vi "Test Digital Input.vi"(8 "error in":errorcluster, 10 "TestCase in":refnum<class "Scan Engine Scripting API Modules.lvclass">, 11 "module test in":refnum<class "Module Test.lvclass">) -> (0 "error out":errorcluster, 2 "TestCase out":refnum<class "Scan Engine Scripting API Modules.lvclass">, 3 "module test out":refnum<class "Module Test.lvclass">)   [LabVIEW 2020, in "Module Test.lvclass"]
uses:
  Module Test.lvclass
  Scan Engine Scripting API Modules.lvclass
  C:/Program Files (x86)/National Instruments/LabVIEW 2020/vi.lib/addons/_JKI Toolkits/VI Tester/TestCase.llb/TestCase.lvclass
  Scripting/Modules/Mode Classes/Controls/digital channel settings.ctl
  Module Test.lvclass/Module Test.ctl
  Scripting/Scan Engine Scripting.lvlib
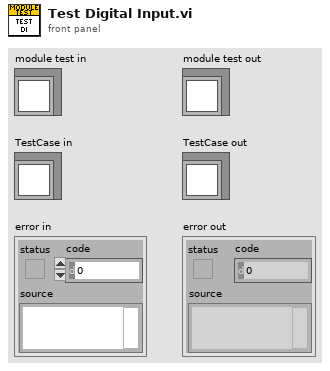
[diagram p1: front panel]
types:
  T1 = typedef "Scan Engine Scripting.lvlib/digital channel settings.ctl" = cluster{"name":string, "default value":bool}
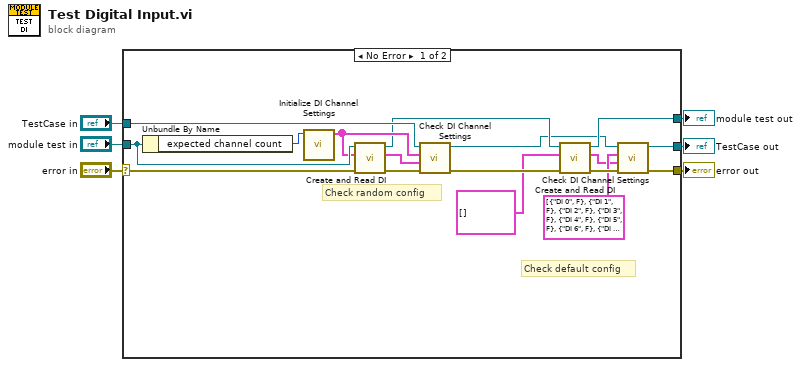
[diagram p0: block diagram]
diagram:
  n1 = case shown="No Error" "error in" {
    selector: "error in" -> [w19 w26]
    tunnel: [w12 w26] -> w5
    tunnel: [w13 w25] -> w3
    tunnel: "module test in" -> [w22 w25]
    tunnel: "TestCase in" -> [w21 w24]
    tunnel: [w9 w24] -> w1
    frame No Error {
      # "Check default config"
      # "Check random config"
      n2 = Unbundle By Name(w22) -> ("expected channel count"=w23:i32)
      n3 = call "Initialize DI Channel Settings.vi"("array size"=w23) -> ("channel settings"=w20:T1[])  [unwired: 10 in]
      n4 = call-dynamic "Create and Read DI.vi"("error in"=w19, "initial channel settings"=w20, "module test in"=w22) -> ("error out"=w18:errorcluster, "read channel settings"=w17:T1[], "module test out"=w16:refnum<class "Module Test.lvclass">)  [unwired: 6 in]
      n5 = call "Check DI Channel Settings.vi"("error in"=w18, "read channel settings"=w17, "initial channel settings"=w20, "TestCase in"=w21) -> ("error out"=w15:errorcluster, "TestCase out"=w10:refnum<class "Scan Engine Scripting API Modules.lvclass">)  [unwired: 6 in]
      n6 = call-dynamic "Create and Read DI.vi"("error in"=w15, "initial channel settings"=T1[] [], "module test in"=w16) -> ("error out"=w11:errorcluster, "read channel settings"=w7:T1[], "module test out"=w13:refnum<class "Module Test.lvclass">)  [unwired: 6 in]
      n7 = call "Check DI Channel Settings.vi"("error in"=w11, "read channel settings"=w7, "initial channel settings"=T1[] [{"name"="DI 0", "default value"=FALSE}, {"name"="DI 1", "default value"=FALSE}, {"name"="DI 2", "default value"=FALSE}, {"name"="DI 3", "default value"=FALSE}, {"name"="DI 4", "default value"=FALSE}, {"name"="DI 5", "default value"=FALSE}, {"name"="DI 6", "default value"=FALSE}, {"name"="DI 7", "default value"=FALSE}], "TestCase in"=w10) -> ("error out"=w12:errorcluster, "TestCase out"=w9:refnum<class "Scan Engine Scripting API Modules.lvclass">)  [unwired: 6 in]
    }
    frame Error {
    }
  }
  "error out" <- w5
  "module test out" <- w3
  "TestCase out" <- w1
